vi "Main Example.vi"() -> ()   [LabVIEW 2014]
uses:
  Stickman State.ctl
  <vilib>/Utility/inputDevices.llb/keyboardAcquire.vi
  <vilib>/Utility/inputDevices.llb/closeKeyboard.vi
panel:
  in  "End Display":bool
  out "Animation Container":picture
  # "For Windows Machines"
  # "2D Image Animation with LabVIEW"
  # "By iterating through arrays of images, you can use LabVIEW to perform image animation. This is easily done for a simple sprite, but what if you wanted your sprite to have more than one kind of action? This is where modular programming comes into play.\n\nPress RIGHT to control \nMr. Stickman."
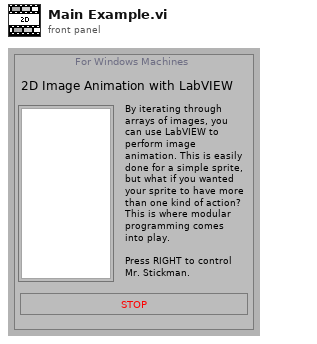
[diagram p1: front panel]
types:
  T1 = typedef "Stickman State.ctl" = enum16{"Standing", "Walking"}
  T2 = enum16{"0", "1", "2", "3", "4", "5", "6", "7", "8", "9", "A", "B", "C", "D", "E", "F", "G", "H", "I", "J", "K", "L", "M", "N", "O", "P", "Q", "R", "S", "T", "U", "V", "W", "X", "Y", "Z", "F1", "F2", "F3", "F4", "F5", "F6", "F7", "F8", "F9", "F10", "F11", "F12", "F13", "F14", "F15", "ADD", "BACK", "BACKSLASH", "CAPITAL", "COMMA", "DECIMAL", "DELETE", "DIVIDE", "DOWN", "END", "EQUALS", "ESCAPE", "GRAVE (`)", "HOME", "INSERT", "LBRACKET", "LCONTROL", "LEFT", "L ALT", "LSHIFT", "LWIN", "MINUS", "MULTIPLY", "NEXT", "NUMLOCK", "NUMPAD_0", "NUMPAD_1", "NUMPAD_2", "NUMPAD_3", "NUMPAD_4", "NUMPAD_5", "NUMPAD_6", "NUMPAD_7", "NUMPAD_8", "NUMPAD_9", "PAUSE", "PERIOD", "PRIOR (PG UP)", "RBRACKET", "RCONTROL", "RETURN", "RIGHT", "R ALT", "RSHIFT", "RWIN", "SCROLL", "SEMICOLON", "SLASH", "SPACE", "SUBTRACT", "TAB", "UP", "ENTER (num pad)", "' (quote)"}[]
  T3 = enum16{"0", "1", "2", "3", "4", "5", "6", "7", "8", "9", "A", "B", "C", "D", "E", "F", "G", "H", "I", "J", "K", "L", "M", "N", "O", "P", "Q", "R", "S", "T", "U", "V", "W", "X", "Y", "Z", "F1", "F2", "F3", "F4", "F5", "F6", "F7", "F8", "F9", "F10", "F11", "F12", "F13", "F14", "F15", "ADD", "BACK", "BACKSLASH", "CAPITAL", "COMMA", "DECIMAL", "DELETE", "DIVIDE", "DOWN", "END", "EQUALS", "ESCAPE", "GRAVE (`)", "HOME", "INSERT", "LBRACKET", "LCONTROL", "LEFT", "L ALT", "LSHIFT", "LWIN", "MINUS", "MULTIPLY", "NEXT", "NUMLOCK", "NUMPAD_0", "NUMPAD_1", "NUMPAD_2", "NUMPAD_3", "NUMPAD_4", "NUMPAD_5", "NUMPAD_6", "NUMPAD_7", "NUMPAD_8", "NUMPAD_9", "PAUSE", "PERIOD", "PRIOR (PG UP)", "RBRACKET", "RCONTROL", "RETURN", "RIGHT", "R ALT", "RSHIFT", "RWIN", "SCROLL", "SEMICOLON", "SLASH", "SPACE", "SUBTRACT", "TAB", "UP", "ENTER (num pad)", "' (quote)"}
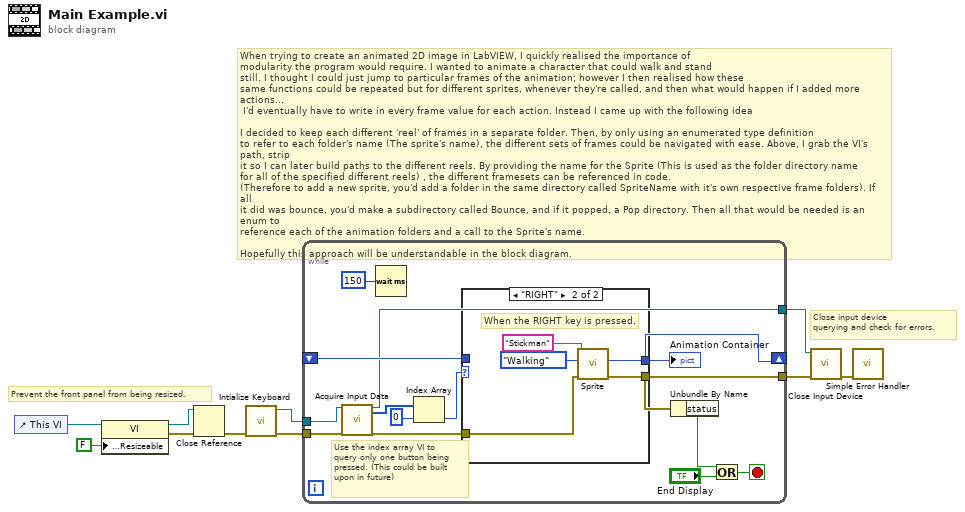
[diagram p0: block diagram]
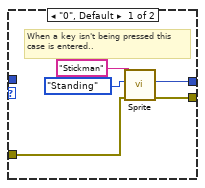
[diagram p2: hidden frame]
diagram:
  # "Close input device\nquerying and check for errors."
  # "Prevent the front panel from being resized."
  # "When trying to create an animated 2D image in LabVIEW, I quickly realised the importance of \nmodularity the program would require. I wanted to animate a character that could walk and stand\nstill. I thought I could just jump to particular frames of the animation; however I then realised how these\nsame functions could be repeated but for different sprites, whenever they're called, and then what would happen if I added more actions...\n I'd eventually have to write in every frame value for each action. Instead I came up with the following idea\n\nI decided to keep each different 'reel' of frames in a separate folder. Then, by only using an enumerated type definition\nto refer to each folder's name (The sprite's name), the different sets of frames could be navigated with ease. Above, I grab the VI's path, strip\nit so I can later build paths to the different reels. By providing the name for the Sprite (This is used as the folder directory name\nfor all of the specified different reels) , the different framesets can be referenced in code.\n(Therefore to add a new sprite, you'd add a folder in the same directory called SpriteName with it's own respective frame folders). If all\nit did was bounce, you'd make a subdirectory called Bounce, and if it popped, a Pop directory. Then all that would be needed is an enum to \nreference each of the animation folders and a call to the Sprite's name. \n\nHopefully this approach will be understandable in the block diagram."
  n1 = control-ref of="This VI"() -> (w5:refnum<vi>)
  n2 = property class="VI"(reference=w5, "Front Panel.Resizeable"=FALSE ("Front Panel Window:Resizable")) -> (reference out=w2:refnum<vi>, error out=w3:errorcluster)  [unwired: 1 in]
  n3 = Close Reference(reference=w2, error in (no error)=w3) -> (error out=w1:errorcluster)
  n4 = call <vilib>:"Intialize Keyboard.vi"("error in (no error)"=w1) -> ("error out"=w9:errorcluster, "device ID"=w10:refnum<k1>)  [unwired: 9 in]
  n5 = while {
    shift-right: [w11] -> _
    shift-left: _ -> [w24]
    tunnel: w10 -> [w23]
    tunnel: w9 -> [w22]
    tunnel: [w18] -> w8
    tunnel: [w15] -> w7
    stop <- w14 stop-if-true
    # "Use the index array VI to\nquery only one button being\npressed. (This could be built\nupon in future)"
    n6 = call-poly <vilib>:"Acquire Input Data.vi"("device ID"=w23, "error in (no error)"=w22) -> ("device ID"=w18:refnum<k1>, "keys pressed"=w21:T2, "error out"=w17:errorcluster)  [unwired: 15 in]
    n7 = Wait (ms)(milliseconds to wait=u32 150) -> ()  [unwired: 1 out]
    n8 = Index Array(array=w21, index=0) -> (element=w19:T3)
    n9 = case shown="\"RIGHT\"" w19 {
      tunnel: [w26 w34] -> w11
      tunnel: w24 -> [_ _]
      tunnel: w17 -> [w29 w32]
      tunnel: [w28 w31] -> w15
      frame "0", Default {
        # "When a key isn't being pressed this\ncase is entered.."
        n10 = call "Sprite.vi"("error in (no error)"=w29, "Sprite Sequence"=Stickman_State."Standing", "Sprite Name"="Stickman") -> ("error out"=w28:errorcluster, "Frame Output"=w26:picture)  [unwired: 5 in, 2 out]
      }
      frame "RIGHT" {
        # "When the RIGHT key is pressed."
        n11 = call "Sprite.vi"("error in (no error)"=w32, "Sprite Sequence"=Stickman_State."Walking" ("Stickman State"), "Sprite Name"="Stickman") -> ("error out"=w31:errorcluster, "Frame Output"=w34:picture)  [unwired: 5 in, 2 out]
      }
    }
    "Animation Container" <- w11
    n12 = Unbundle By Name(w15) -> ("status"=w12:bool)
    n13 = Or(x=w12, y="End Display") -> (x .or. y?=w14:bool)
  }
  n14 = call-poly <vilib>:"Close Input Device.vi"("error in (no error)"=w7, "device ID"=w8) -> ("error out"=w6:errorcluster)  [unwired: 8 in]
  n15 = call <vilib>:"Simple Error Handler.vi"("error in (no error)"=w6) -> ()  [unwired: 4 in, 5 out]
